vi "Sub_get_freq_bounds_FEA.vi"(0 "Setup Parameters":T2, 1 "LEMP":T3) -> (2 "Beam frequency params":T1 {"Max frequency delta per node" format="%0.2f"}, 3 "cross over":i32, 4 "nodes of interest":i32[](array[numeric]), 5 "all nodes":i32[](array[numeric]))   [LabVIEW 2021]
panel:
  out "third modes":dbl[](array[numeric])
  out "first modes":dbl[](array[numeric])
  out "second modes":dbl[](array[numeric])
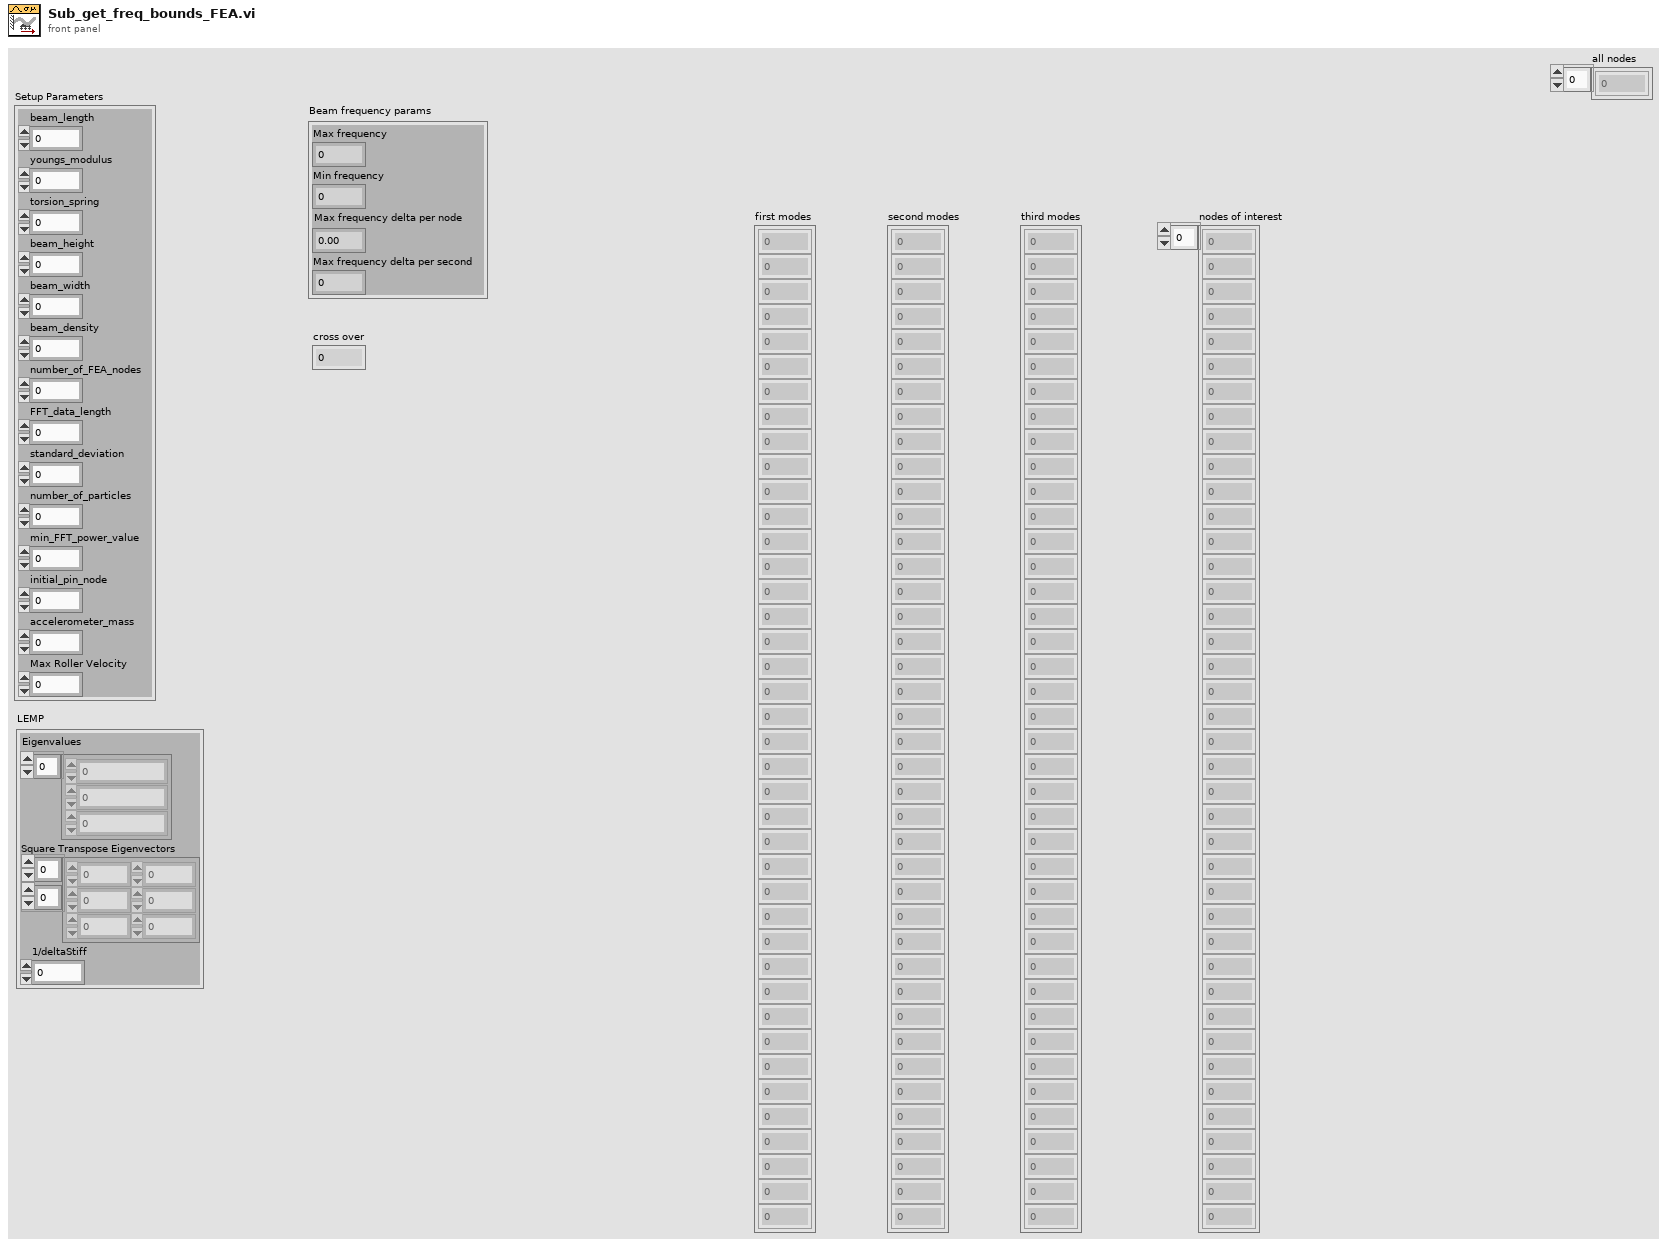
[diagram p1: front panel]
types:
  T1 = cluster{"Max frequency":dbl, "Min frequency":dbl, "Max frequency delta per node":dbl, "Max frequency delta per second":dbl}
  T2 = cluster{"beam_length":dbl, "youngs_modulus":dbl, "torsion_spring":dbl, "beam_height":dbl, "beam_width":dbl, "beam_density":dbl, "number_of_FEA_nodes":i32, "FFT_data_length":i32, "standard_deviation":dbl, "number_of_particles":i32, "min_FFT_power_value":dbl, "initial_pin_node":i32, "accelerometer_mass":dbl, "Max Roller Velocity":dbl}
  T3 = cluster{"Eigenvalues":dbl[], "Square Transpose Eigenvectors":dbl[][], "1/deltaStiff":dbl}
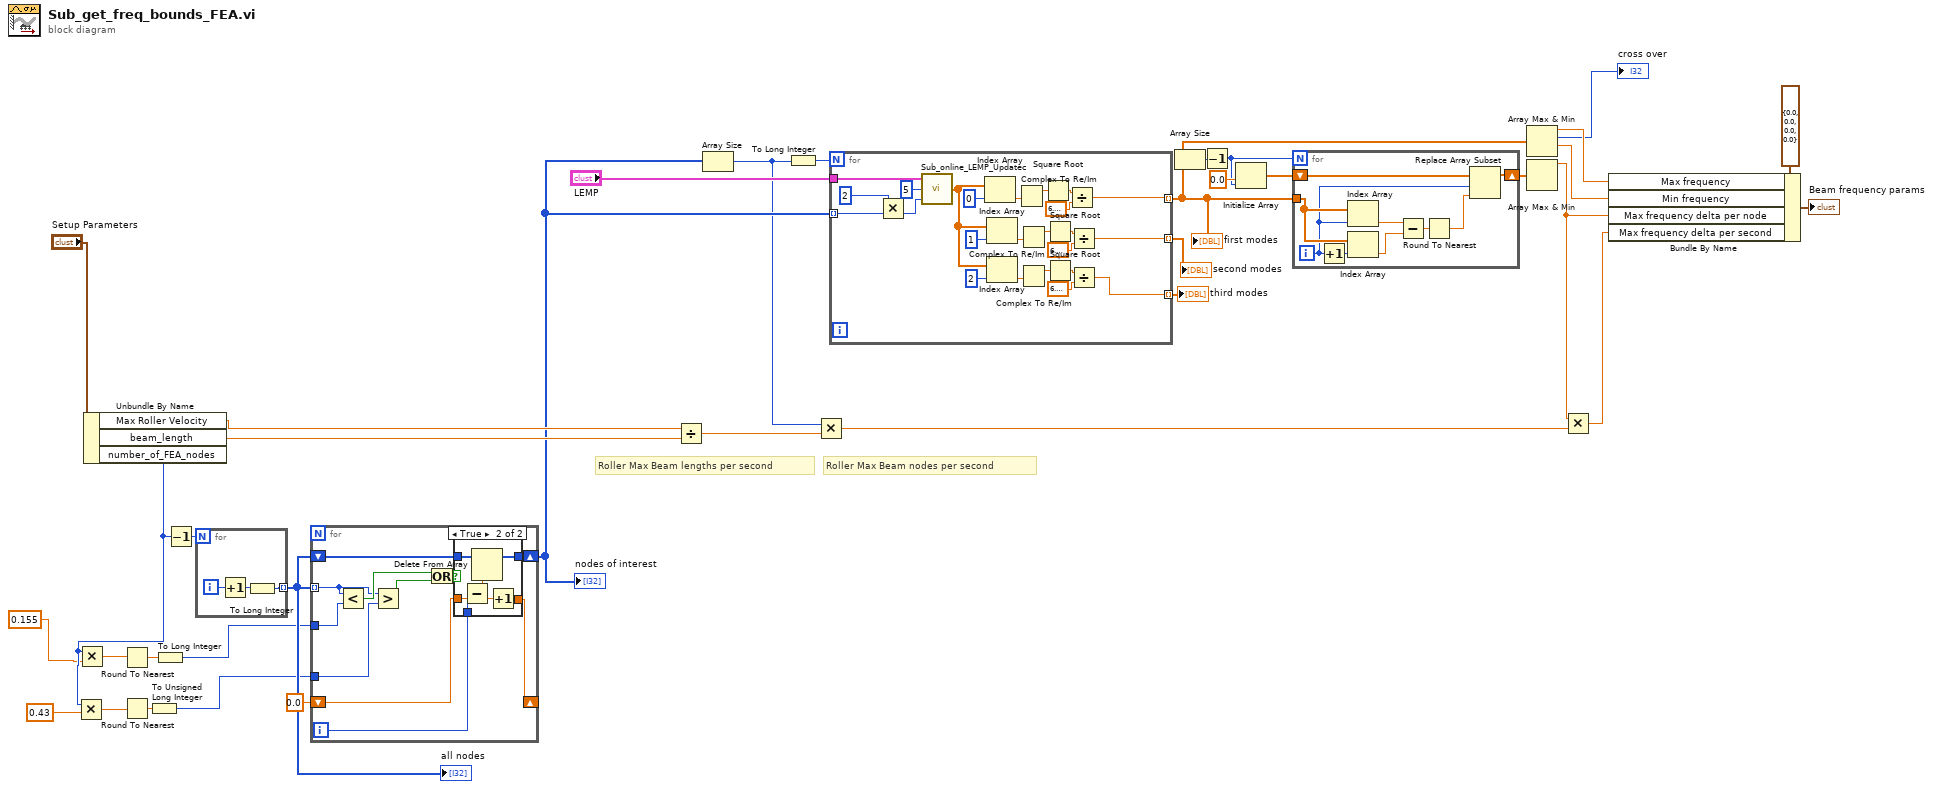
[diagram p0: block diagram]
diagram:
  # "Roller Max Beam nodes per second"
  # "Roller Max Beam lengths per second"
  n1 = Unbundle By Name("Setup Parameters") -> ("Max Roller Velocity"=w27:dbl, "beam_length"=w26:dbl, "number_of_FEA_nodes"=w8:i32)
  n2 = Multiply(x=w8, y=0.43) -> (x*y=w7:dbl)
  n3 = Multiply(x=w8, y=0.155) -> (x*y=w6:dbl)
  n4 = Round To Nearest(number=w6) -> (nearest integer value=w5:dbl)
  n5 = Round To Nearest(number=w7) -> (nearest integer value=w4:dbl)
  n6 = To Unsigned Long Integer(number=w4) -> (unsigned 32bit integer=w3:u32)
  n7 = To Long Integer(number=w5) -> (32bit integer=w2:i32)
  n8 = Decrement(x=w8) -> (x-1=w15:i32)
  n9 = for {
    N: w15 -> [_]
    tunnel: [w39] -> w14 mode=indexing
    i -> [w37]
    n10 = Increment(x=w37) -> (x+1=w38:i32)
    n11 = To Long Integer(number=w38) -> (32bit integer=w39:i32)
  }
  "all nodes" <- w14
  n12 = for {
    tunnel: w14 -> [w43] mode=indexing
    shift-right: [w46] -> w11
    shift-left: w14 -> [w50]
    shift-right: [w45] -> _
    shift-left: 0.0 -> [w44]
    tunnel: w2 -> [w41]
    tunnel: w3 -> [w40]
    i -> [w42]
    n13 = Less?(x=w43, y=w41) -> (x < y?=w47:bool)
    n14 = Greater?(x=w43, y=w40) -> (0:w49:bool)
    n15 = Or(x=w47, y=w49) -> (x .or. y?=w48:bool)
    n16 = case shown="True" w48 {
      tunnel: w50 -> [w52 w57]
      tunnel: [w52 w58] -> w46
      tunnel: [w51 w56] -> w45
      tunnel: w44 -> [w51 w55]
      tunnel: w42 -> [_ w54]
      frame False {
      }
      frame True {
        n17 = Subtract(x=w54, y=w55) -> (x-y=w53:dbl)
        n18 = Delete From Array(array=w57, index=w53) -> (array with subset deleted=w58:i32[])  [unwired: 1 in, 1 out]
        n19 = Increment(x=w55) -> (x+1=w56:dbl)
      }
    }
  }
  "nodes of interest" <- w11
  n20 = Divide(x=w27, y=w26) -> (x/y=w29:dbl)
  n21 = Array Size(array=w11) -> (size(s)=w10:i32)
  n22 = To Long Integer(number=w10) -> (32bit integer=w18:i32)
  n23 = Multiply(x=w10, y=w29) -> (x*y=w28:dbl)
  n24 = for {
    N: w18 -> [_]
    tunnel: "LEMP" -> [w80]
    tunnel: [w73] -> w34 mode=indexing
    tunnel: [w67] -> w17 mode=indexing
    tunnel: [w60] -> w16 mode=indexing
    tunnel: w11 -> [w59] mode=indexing
    n25 = Multiply(x=2, y=w59) -> (x*y=w79:i32)
    n26 = call "Sub_online_LEMP_Updatec.vi"("Effected DOF"=w79, "Mode count"=5, "LEMP"=w80) -> ("Updated Eigenvalues"=w61:dbl[])
    n27 = Index Array(array=w61, index=0) -> (element=w77:dbl)
    n28 = Index Array(array=w61, index=1) -> (element=w72:dbl)
    n29 = Index Array(array=w61, index=2) -> (element=w66:dbl)
    n30 = Complex To Re/Im(x + iy=w77) -> (x=w76:dbl)  [unwired: 1 out]
    n31 = Complex To Re/Im(x + iy=w72) -> (x=w71:dbl)  [unwired: 1 out]
    n32 = Complex To Re/Im(x + iy=w66) -> (x=w65:dbl)  [unwired: 1 out]
    n33 = Square Root(x=w76) -> (sqrt(x)=w75:dbl)
    n34 = Square Root(x=w71) -> (sqrt(x)=w70:dbl)
    n35 = Square Root(x=w65) -> (sqrt(x)=w64:dbl)
    n36 = Divide(x=w75, y=6.283185307179586) -> (x/y=w73:dbl)
    n37 = Divide(x=w70, y=6.283185307179586) -> (x/y=w67:dbl)
    n38 = Divide(x=w64, y=6.283185307179586) -> (x/y=w60:dbl)
  }
  "second modes" <- w17
  "first modes" <- w34
  "third modes" <- w16
  n39 = Array Size(array=w34) -> (size(s)=w35:i32)
  n40 = Decrement(x=w35) -> (x-1=w31:i32)
  n41 = Initialize Array(0.0 ("element"), w31) -> (w33:dbl[])
  n42 = for {
    N: w31 -> [_]
    tunnel: w34 -> [w91]
    shift-right: [w85] -> w30
    shift-left: w33 -> [w86]
    i -> [w84]
    n43 = Increment(x=w84) -> (x+1=w90:i32)
    n44 = Index Array(array=w91, index=w84) -> (element=w89:dbl)
    n45 = Index Array(array=w91, index=w90) -> (element=w88:dbl)
    n46 = Subtract(x=w89, y=w88) -> (x-y=w87:dbl)
    n47 = Round To Nearest(number=w87) -> (nearest integer value=w83:dbl)
    n48 = Replace Array Subset(array=w86, new element=w83, index=w84) -> (w85:dbl[])
  }
  n49 = Array Max & Min(array=w34) -> (max value=w20:dbl, max index (indices)=→"cross over":i32, min value=w23:dbl)  [unwired: 1 out]
  n50 = Array Max & Min(array=w30) -> (max value=w21:dbl)  [unwired: 3 out]
  n51 = Multiply(x=w21, y=w28) -> (x*y=w22:dbl)
  n52 = Bundle By Name(cluster=T1 {"Max frequency"=0.0, "Min frequency"=0.0, "Max frequency delta per node"=0.0, "Max frequency delta per second"=0.0} ("Beam frequency params"), "Max frequency"=w20, "Min frequency"=w23, "Max frequency delta per node"=w21, "Max frequency delta per second"=w22) -> (→"Beam frequency params":T1)
